vi "Data_Uniform Square.vi"(6 "seed":i32=-1, 10 "amplitude":dbl=1.0 format="%0.2f", 11 "# of points":i32=4000) -> (1 "Classes":i32[](array[numeric]), 3 "Data":dbl[][](array[numeric]))   [LabVIEW 2009]
uses:
  <vilib>/Analysis/NI_AALBase.lvlib
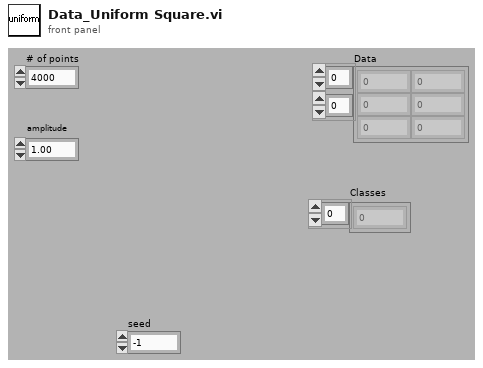
[diagram p1: front panel]
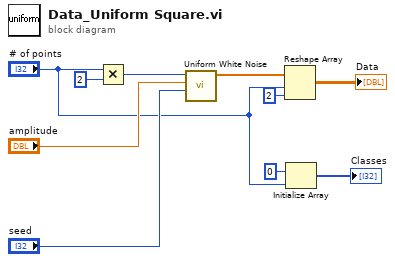
[diagram p0: block diagram]
diagram:
  n1 = Multiply(x="# of points", y=2) -> (x*y=w9:i32)
  n2 = call <vilib>:"Uniform White Noise.vi"("seed"="seed", "amplitude"="amplitude", "samples"=w9) -> ("uniform white noise"=w6:dbl[])  [unwired: 7 in, 1 out]
  n3 = Reshape Array(w6, "# of points", 2 ("dimension size")) -> (→"Data":dbl[][])
  n4 = Initialize Array(0 ("element"), "# of points") -> (→"Classes":i32[])
